vi "Graph 3.vi"() -> ()   [LabVIEW 2024]
panel:
  out "XY Graph 2":cluster{dbl[], dbl[]}[](graph)
  out "XY Graph":cluster{"X":dbl, "Y":dbl}[](graph)
  out "Waveform Chart":cluster{dbl, dbl}(graph)
  in  "stop":bool
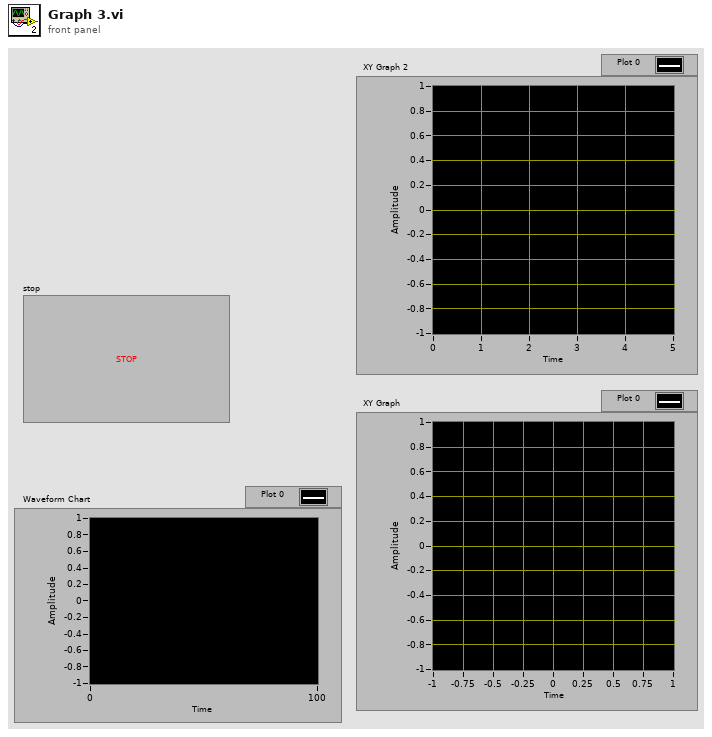
[diagram p1: front panel]
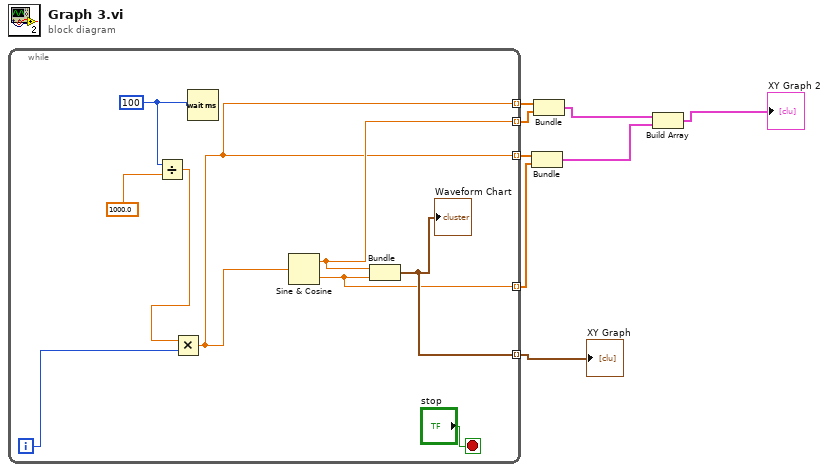
[diagram p0: block diagram]
diagram:
  n1 = while {
    tunnel: [w12] -> w8 mode=indexing
    tunnel: [w10] -> w7 mode=indexing
    tunnel: [w11] -> w6 mode=indexing
    tunnel: [w10] -> w5 mode=indexing
    tunnel: [w9] -> w4 mode=indexing
    i -> [w14]
    stop <- "stop" stop-if-true
    w15 = u32 100 ("milliseconds to wait")
    n2 = Divide(x=w15, y=1000.0) -> (x/y=w13:dbl)
    n3 = Multiply(x=w13, y=w14) -> (x*y=w10:dbl)
    n4 = Wait (ms)(milliseconds to wait=w15) -> ()  [unwired: 1 out]
    n5 = Sine & Cosine(0:w10) -> (1:w11:dbl, 2:w9:dbl)
    n6 = Bundle(w11, w9) -> (w12:cluster{dbl, dbl})  [unwired: 1 in]
    "Waveform Chart" <- w12
  }
  "XY Graph" <- w8
  n7 = Bundle(w5, w4) -> (w2:cluster{dbl[], dbl[]})  [unwired: 1 in]
  n8 = Bundle(w7, w6) -> (w3:cluster{dbl[], dbl[]})  [unwired: 1 in]
  n9 = Build Array(w3, w2) -> (→"XY Graph 2":cluster{dbl[], dbl[]}[])
